vi "Coerce Y Output Waveform.vi"(1 "X Output Waveform":waveform(dbl)) -> (0 "Coerced X Output Waveform":waveform(dbl))   [LabVIEW 2013]
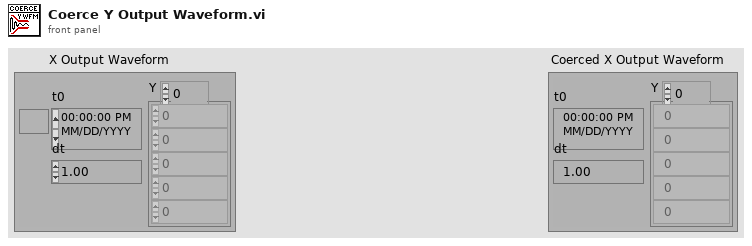
[diagram p1: front panel]
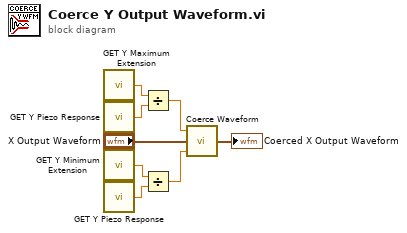
[diagram p0: block diagram]
diagram:
  n1 = call "GET Y Maximum Extension.vi"() -> ("Y Maximum Extension"=w6:dbl)
  n2 = call "GET Y Piezo Response.vi"() -> ("Y Piezo Response"=w5:dbl)
  n3 = call "GET Y Minimum Extension.vi"() -> ("Y Minimum Extension"=w3:dbl)
  n4 = call "GET Y Piezo Response.vi"() -> ("Y Piezo Response"=w2:dbl)
  n5 = Divide(x=w6, y=w5) -> (x/y=w1:dbl)
  n6 = Divide(x=w3, y=w2) -> (x/y=w4:dbl)
  n7 = call "Coerce Waveform.vi"("Lower Limit"=w4, "Output Waveform"="X Output Waveform", "Upper Limit"=w1) -> ("Coerced Output Waveform"=→"Coerced X Output Waveform":waveform(dbl))
